vi "Droite_Panneau.vi"() -> ()   [LabVIEW 2023]
uses:
  <vilib>/Utility/miscctls.llb/LVRectTypeDef.ctl
  <vilib>/Utility/miscctls.llb/LVBoundsTypeDef.ctl
  <vilib>/Utility/miscctls.llb/LVPointTypeDef.ctl
panel:
  out "Width 3":u32
  out "Width 2":u32
  out "Width":u32
  out "Ep Barre":u32
  out "Booléen 2":bool
  in  "Lect/Ecr Pos Barre":bool
  out "épaisseur barre":u32
  out "Delta F":i16
  out "Limites":T1
  in  "stop":bool
  out "Fenêtre face-avant:Limites face-avant":T2
  in  "Commande onglets":enum32{"Page 1", "Page 2"}(tab)
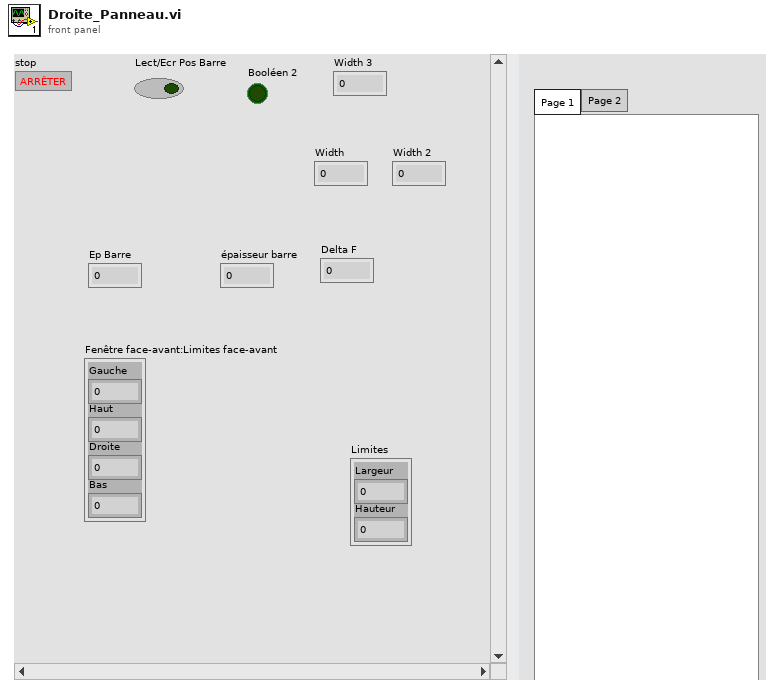
[diagram p1: front panel]
types:
  T1 = typedef "LVBoundsTypeDef.ctl" = cluster{"Width":u32, "Height":u32}
  T2 = typedef "LVRectTypeDef.ctl" = cluster{"Left":i16, "Top":i16, "Right":i16, "Bottom":i16}
  T3 = typedef "LVPointTypeDef.ctl" = cluster{"Horizontal":i16, "Vertical":i16}
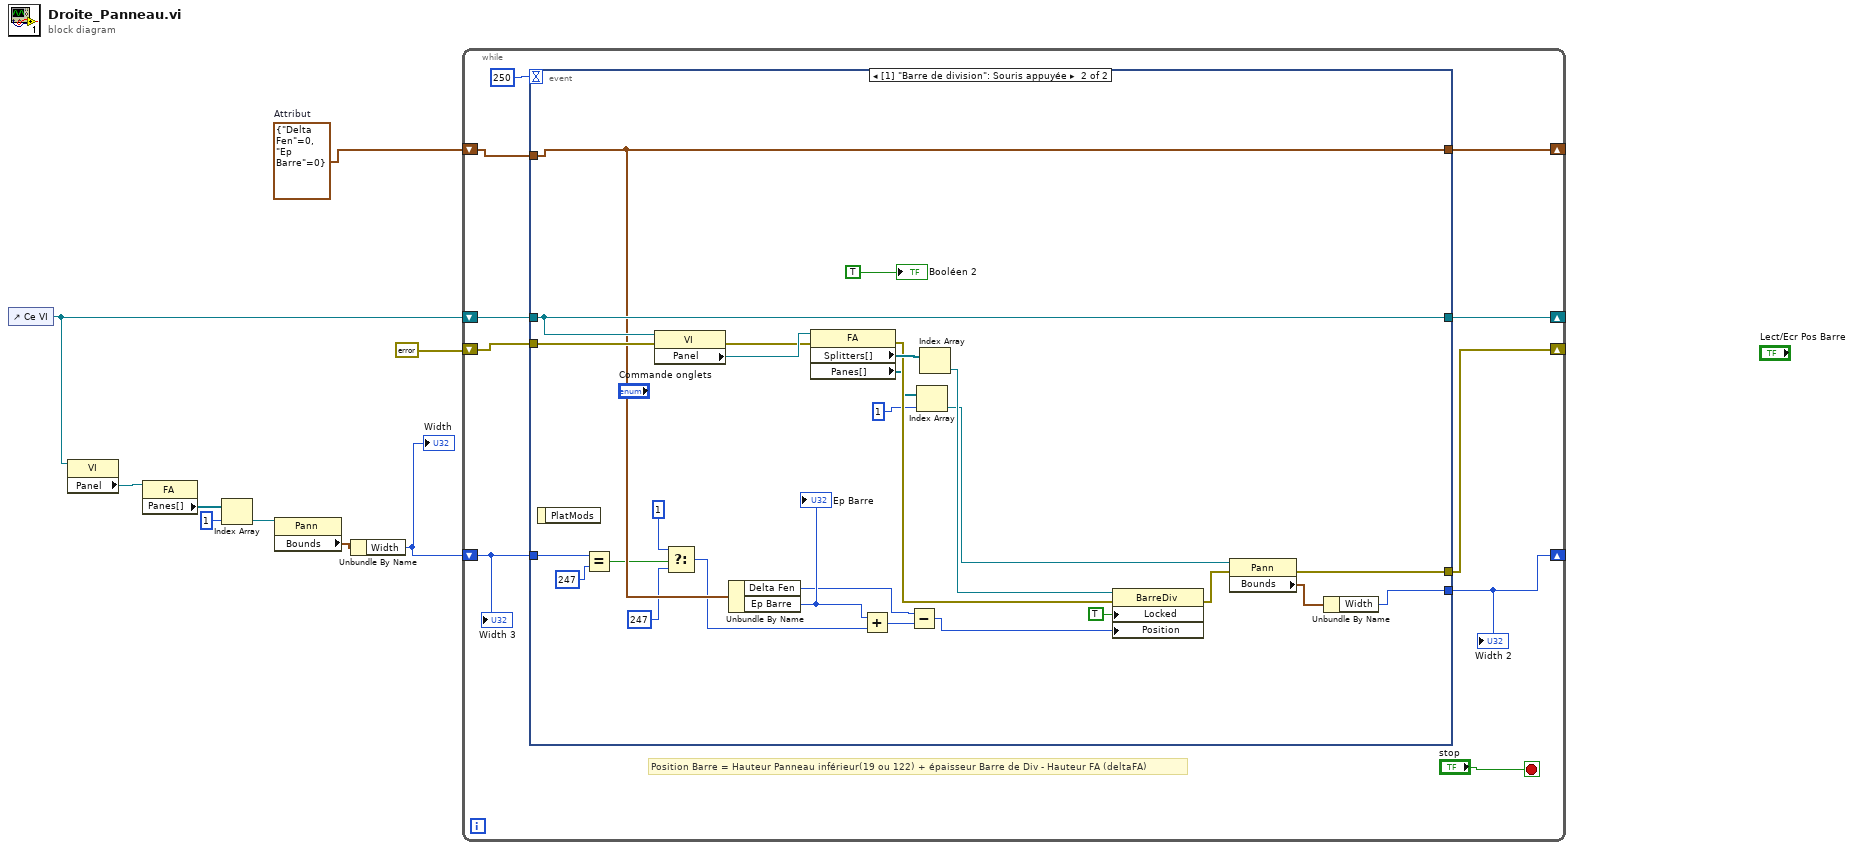
[diagram p0: block diagram]
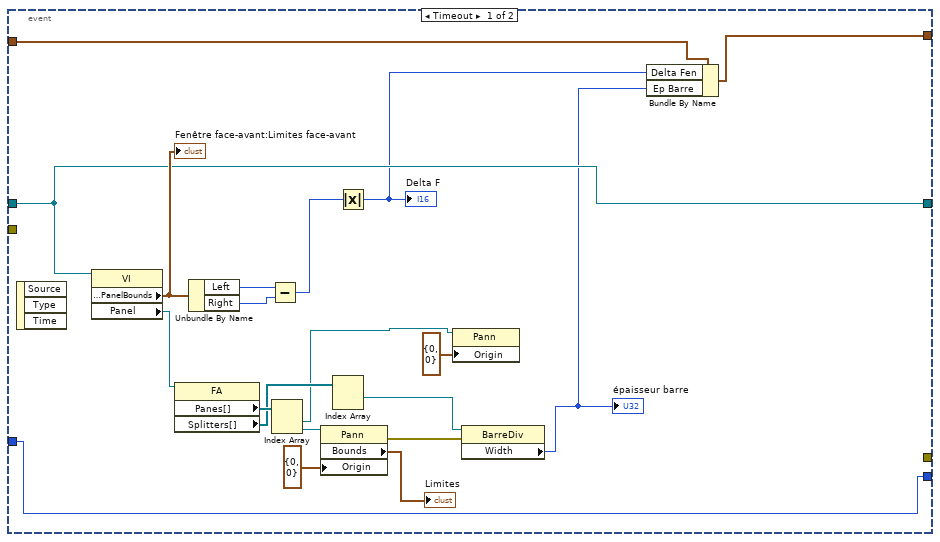
[diagram p2: hidden frame]
diagram:
  w8 = cluster{"Delta Fen":i16, "Ep Barre":u32} {"Delta Fen"=0, "Ep Barre"=0}  # Attribut
  n1 = control-ref of="Ce VI"() -> (w7:refnum<vi>)
  n2 = property class="VI"(reference=w7) -> ("Panel"=w6:refnum<vi>)  [unwired: 1 in, 2 out]
  n3 = property class="FA"(reference=w6) -> ("Panes[]"=w5:refnum<vi>[])  [unwired: 1 in, 2 out]
  n4 = Index Array(array=w5, index=1 ("indice")) -> (element=w3:refnum<vi>)
  n5 = property class="Pann"(reference=w3) -> ("Bounds"=w2:T1)  [unwired: 1 in, 2 out]
  n6 = Unbundle By Name(w2) -> ("Width"=w1:u32)
  "Width" <- w1
  n7 = while {
    shift-right: [w16] -> _
    shift-left: w7 -> [w18]
    shift-right: [w15] -> _
    shift-left: errorcluster {"status"=FALSE, "code"=0, "source"=""} ("error out") -> [w14]
    shift-right: [w13] -> _
    shift-left: w8 -> [w12]
    shift-right: [w11] -> _
    shift-left: w1 -> [w10]
    stop <- "stop" stop-if-true
    # "Position Barre = Hauteur Panneau inférieur(19 ou 122) + épaisseur Barre de Div - Hauteur FA (deltaFA)"
    n8 = event shown="[1] \"Barre de division\": Souris appuyée" {
      selector: _ -> [_ _]
      dyn-events: _ -> [_ _]
      timeout: 250 -> [_ _]
      tunnel: w18 -> [w26 w62]
      tunnel: [w26 w62] -> w16
      tunnel: [_ w47] -> w15
      tunnel: w14 -> [_ w63]
      tunnel: [w21 w59] -> w13
      tunnel: w12 -> [w24 w59]
      tunnel: w10 -> [w20 w49]
      tunnel: [w20 w50] -> w11
      event Timeout {
        n9 = event-data() -> ()  [unwired: 1 in, 3 out]
        n10 = property class="VI"(reference=w26) -> ("Front Panel.PanelBounds"=w30:T2, "Panel"=w39:refnum<vi>)  [unwired: 1 in, 2 out]
        "Fenêtre face-avant:Limites face-avant" <- w30
        n11 = property class="FA"(reference=w39) -> ("Panes[]"=w38:refnum<vi>[], "Splitters[]"=w33:refnum<vi>[])  [unwired: 1 in, 2 out]
        n12 = Unbundle By Name(w30) -> ("Left"=w29:i16, "Right"=w28:i16)
        n13 = Subtract(x=w29, y=w28) -> (x-y=w27:i16)
        n14 = Index Array(array=w38) -> (element #1=w31:refnum<vi>, element #2=w37:refnum<vi>)  [unwired: 2 in]
        n15 = property class="Pann"(reference=w37, "Origin"=T3 {"Horizontal"=0, "Vertical"=0} ("Origine")) -> (error out=w34:errorcluster, "Bounds"=→"Limites":T1)  [unwired: 1 in, 1 out]
        n16 = Index Array(array=w33) -> (element #1=w32:refnum<vi>)  [unwired: 2 in, 1 out]
        n17 = Absolute Value(x=w27) -> (abs(x)=w23:i16)
        "Delta F" <- w23
        n18 = property class="Pann"(reference=w31, "Origin"=T3 {"Horizontal"=0, "Vertical"=0} ("Origine")) -> ()  [unwired: 1 in, 2 out]
        n19 = property class="BarreDiv"(reference=w32, error in=w34) -> ("Width"=w22:u32)  [unwired: 2 out]
        "épaisseur barre" <- w22
        n20 = Bundle By Name(cluster=w24, "Delta Fen"=w23, "Ep Barre"=w22) -> (w21:cluster{"Delta Fen":i16, "Ep Barre":u32})
      }
      event Mouse Down {
        n21 = event-data() -> ()  [unwired: 1 in, 1 out]
        n22 = Equal?(x=w49, y=u32 247) -> (x = y?=w46:bool)
        n23 = property class="VI"(reference=w62, error in=w63) -> (error out=w64:errorcluster, "Panel"=w66:refnum<vi>)  [unwired: 1 out]
        n24 = Select(t=u32 1 ("y"), s=w46, f=u32 247 ("y")) -> (s? t:f=w48:u32)
        n25 = Unbundle By Name(w59) -> ("Delta Fen"=w57:i16, "Ep Barre"=w58:u32)
        "Ep Barre" <- w58
        n26 = property class="FA"(reference=w66, error in=w64) -> (error out=w55:errorcluster, "Splitters[]"=w65:refnum<vi>[], "Panes[]"=w53:refnum<vi>[])  [unwired: 1 out]
        n27 = Add(x=w58, y=w48) -> (x+y=w60:u32)
        n28 = Subtract(x=w57, y=w60) -> (x-y=w41:u32)
        n29 = Index Array(array=w53, index=1 ("indice")) -> (element=w45:refnum<vi>)
        n30 = Index Array(array=w65) -> (element=w56:refnum<vi>)  [unwired: 1 in]
        n31 = property class="BarreDiv"(reference=w56, error in=w55, "Locked"=TRUE ("Position de barre de division verrouillée"), "Position"=w41) -> (error out=w52:errorcluster)  [unwired: 1 out]
        n32 = property class="Pann"(reference=w45, error in=w52) -> (error out=w47:errorcluster, "Bounds"=w51:T1)  [unwired: 1 out]
        n33 = Unbundle By Name(w51) -> ("Width"=w50:u32)
        "Booléen 2" <- TRUE
      }
    }
    "Width 2" <- w11
    "Width 3" <- w10
  }
